vi "Write AllowUserToResizeColumns.vi"(8 "error in (no error)":errorcluster, 10 "AllowUserToResizeColumns":bool=TRUE, 11 "DataGridView in":refnum<class "DataGridView.lvclass">) -> (0 "error out":errorcluster, 3 "DataGridView out":refnum<class "DataGridView.lvclass">)   [LabVIEW 2013, in "DataGrid.lvlib" / "DataGridView.lvclass"]
uses:
  DataGridView.lvclass
  System.Windows.Forms
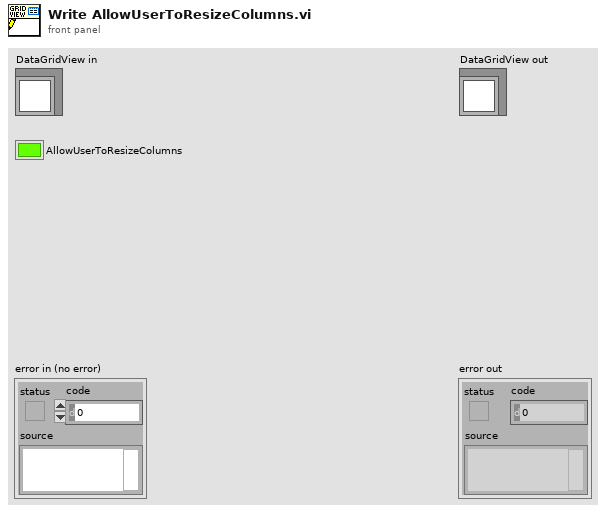
[diagram p1: front panel]
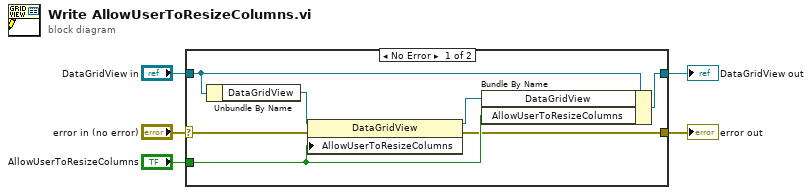
[diagram p0: block diagram]
diagram:
  n1 = case shown="No Error" "error in (no error)" {
    selector: "error in (no error)" -> [w8 w13]
    tunnel: [w7 w13] -> w4
    tunnel: [w12 w14] -> w2
    tunnel: "DataGridView in" -> [w11 w14]
    tunnel: "AllowUserToResizeColumns" -> [w10 _]
    frame No Error {
      n2 = Unbundle By Name(w11) -> ("DataGridView"=w9:refnum<k24>)
      n3 = property class="DataGridView"(reference=w9, error in=w8, "AllowUserToResizeColumns"=w10) -> (reference out=w6:refnum<k24>, error out=w7:errorcluster)
      n4 = Bundle By Name(cluster=w11, "DataGridView"=w6, "AllowUserToResizeColumns"=w10) -> (w12:refnum<class "DataGridView.lvclass">)
    }
    frame Error {
    }
  }
  "error out" <- w4
  "DataGridView out" <- w2
